vi "Compile Incoming Frames.vi"(8 "error in (no error)":errorcluster, 10 "Refs":T3[](array[typedef]) {"Signal Refs" format="%.0x"}, 11 "Item Ref in":T2 format="%.0x") -> (0 "error out":errorcluster, 1 "Refs":T1[](array[typedef]) format="%.0x", 2 "Lookup Table":variant, 3 "Item Ref out":T2=18446744073709551615 format="%.0x")   [LabVIEW 2015, in "Diagnostics Addon System Explorer.lvlib"]
uses:
  System Explorer/Diagnostics Addon System Explorer.lvlib
  <vilib>/NI Veristand/Custom Device API/Custom Device Item Ref.ctl
  Frame Signal VS References.ctl
  <vilib>/NI Veristand/Custom Device API/Data Reference.ctl
  <vilib>/NI Veristand/Custom Device API/Data Access Type.ctl
  Datatable Lookup Positions.ctl
  Shared/Diagnostics Addon Shared.lvlib
  <vilib>/NI Veristand/Custom Device API/Custom Device API.lvlib
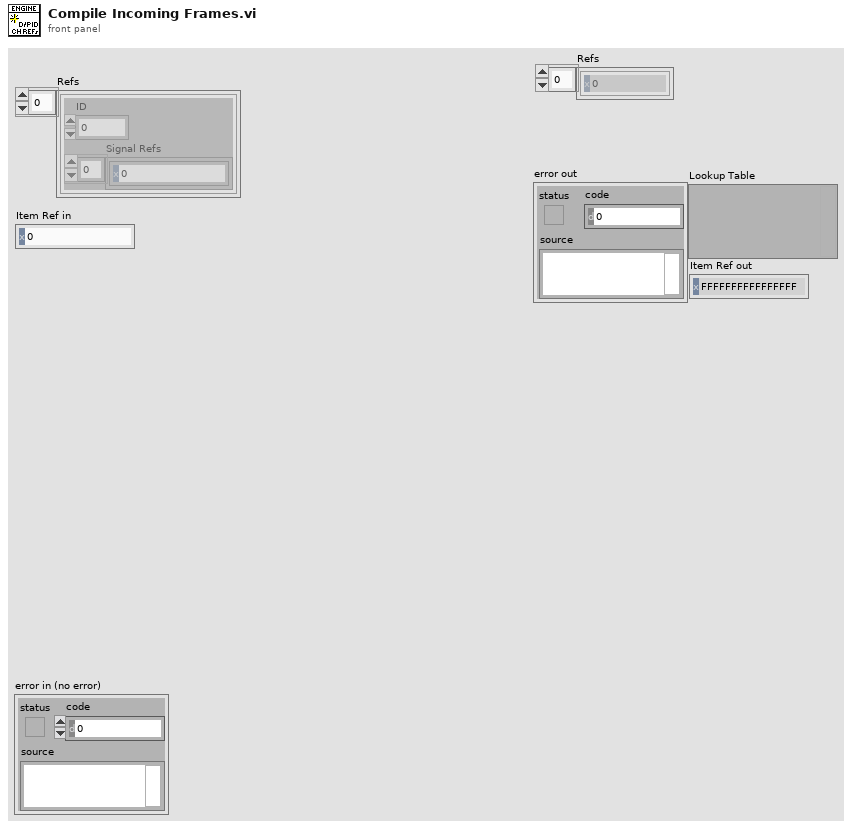
[diagram p1: front panel]
types:
  T1 = typedef "Custom Device API.lvlib/Data Reference.ctl" = i32
  T2 = typedef "Custom Device API.lvlib/Custom Device Item Ref.ctl" = u64
  T3 = typedef "Diagnostics Addon System Explorer.lvlib/Frame Signal VS References.ctl" = cluster{"ID":u16, "Signal Refs":T2[]}
  T4 = typedef "Custom Device API.lvlib/Data Access Type.ctl" = enum16{"Read", "Write"}
  T5 = typedef "Diagnostics Addon Shared.lvlib/Datatable Lookup Positions.ctl" = cluster{"Offset":i32, "Length":i32}
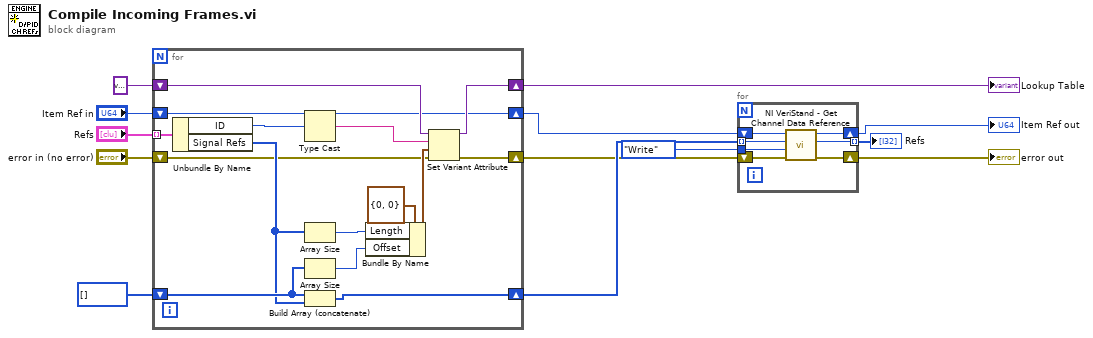
[diagram p0: block diagram]
diagram:
  n1 = for {
    tunnel: "Refs" -> [w18] mode=indexing
    shift-right: [w27] -> w5
    shift-left: T2[] [] ("Signal Refs") -> [w28]
    shift-right: [w19] -> w9
    shift-left: variant -> [w23]
    shift-right: [w21] -> w4
    shift-left: "error in (no error)" -> [w15]
    shift-right: [w14] -> w6
    shift-left: "Item Ref in" -> [w14]
    n2 = Unbundle By Name(w18) -> ("ID"=w17:u16, "Signal Refs"=w16:T2[])
    n3 = Type Cast(x=w17) -> (*(type *) &x=w20:string)  [unwired: 1 in]
    n4 = Array Size(array=w16) -> (size(s)=w26:i32)
    n5 = Array Size(array=w28) -> (size(s)=w22:i32)
    n6 = Build Array (concatenate)(w28, w16) -> (w27:T2[])
    n7 = Bundle By Name(cluster=T5 {"Offset"=0, "Length"=0}, "Length"=w26, "Offset"=w22) -> (w24:T5)
    n8 = Set Variant Attribute(Variant=w23, name=w20, value=w24, error in=w15) -> (Variant out=w19:variant, error out=w21:errorcluster)  [unwired: 1 out]
  }
  "Lookup Table" <- w9
  n9 = for {
    tunnel: w5 -> [w31] mode=indexing
    tunnel: Data_Access_Type."Write" ("Access") -> [w30]
    shift-right: [w33] -> w3
    shift-left: w4 -> [w34]
    shift-right: [w35] -> w2
    shift-left: w6 -> [w32]
    tunnel: [w29] -> w1 mode=indexing
    n10 = call <vilib>:"NI VeriStand - Get Channel Data Reference.vi"("error in (no error)"=w34, "Access"=w30, "Channel Ref in"=w31, "Device Ref in"=w32) -> ("error out"=w33:errorcluster, "Channel Data Reference"=w29:T1, "Device Ref out"=w35:T2)  [unwired: 5 in]
  }
  "error out" <- w3
  "Item Ref out" <- w2
  "Refs" <- w1
